vi "InitDir.vi"(8 "error in":errorcluster, 11 "MainFGV_data in":T1={"TestDir"=path "", "TestName"="", "task"="", "data_file"=refnum, "AcqQueue"=refnum, "StartTime"=timestamp(0 s since 1904-01-01), "config_channels"=[], "DAQmx Device"="", "Advanced"={"rate"=1652.0, "duration"=1.0, "thr"=100.0, "preTrigger"=100.0, "cutoff"=-3.0, "Filtro"=enum."Desativado", "highPass"=1000.0, "lowPass"=1000.0, "updateTime"=50.0}, "running"=FALSE, "hammerIndex"=0, "session"="localhost"} {"Advanced"."updateTime" format="%#_g ms"; "Advanced"."lowPass" format="%#_g Hz"; "Advanced"."highPass" format="%#_g Hz"; "Advanced"."cutoff" format="%#_g dB"; "Advanced"."preTrigger" format="%#_g ms"; "Advanced"."thr" format="%#_g N"; "Advanced"."duration" format="%#_g s"; "Advanced"."rate" min=1652.0 max=51200.0 format="%#_g Hz"}) -> (0 "error out":errorcluster, 3 "MainFGV_data":T1={"TestDir"=path "", "TestName"="", "task"="", "data_file"=refnum, "AcqQueue"=refnum, "StartTime"=timestamp(0 s since 1904-01-01), "config_channels"=[], "DAQmx Device"="", "Advanced"={"rate"=1652.0, "duration"=1.0, "thr"=100.0, "preTrigger"=100.0, "cutoff"=-3.0, "Filtro"=enum."Desativado", "highPass"=1000.0, "lowPass"=1000.0, "updateTime"=50.0}, "running"=FALSE, "hammerIndex"=0, "session"="localhost"} {"Advanced"."updateTime" format="%#_g ms"; "Advanced"."lowPass" format="%#_g Hz"; "Advanced"."highPass" format="%#_g Hz"; "Advanced"."cutoff" format="%#_g dB"; "Advanced"."preTrigger" format="%#_g ms"; "Advanced"."thr" format="%#_g N"; "Advanced"."duration" format="%#_g s"; "Advanced"."rate" min=1652.0 max=51200.0 format="%#_g Hz"})   [LabVIEW 2016]
uses:
  MainFGV_data.ctl
  Settings/config_board.ctl
  Settings/Advanced/AdvancedConfig.ctl
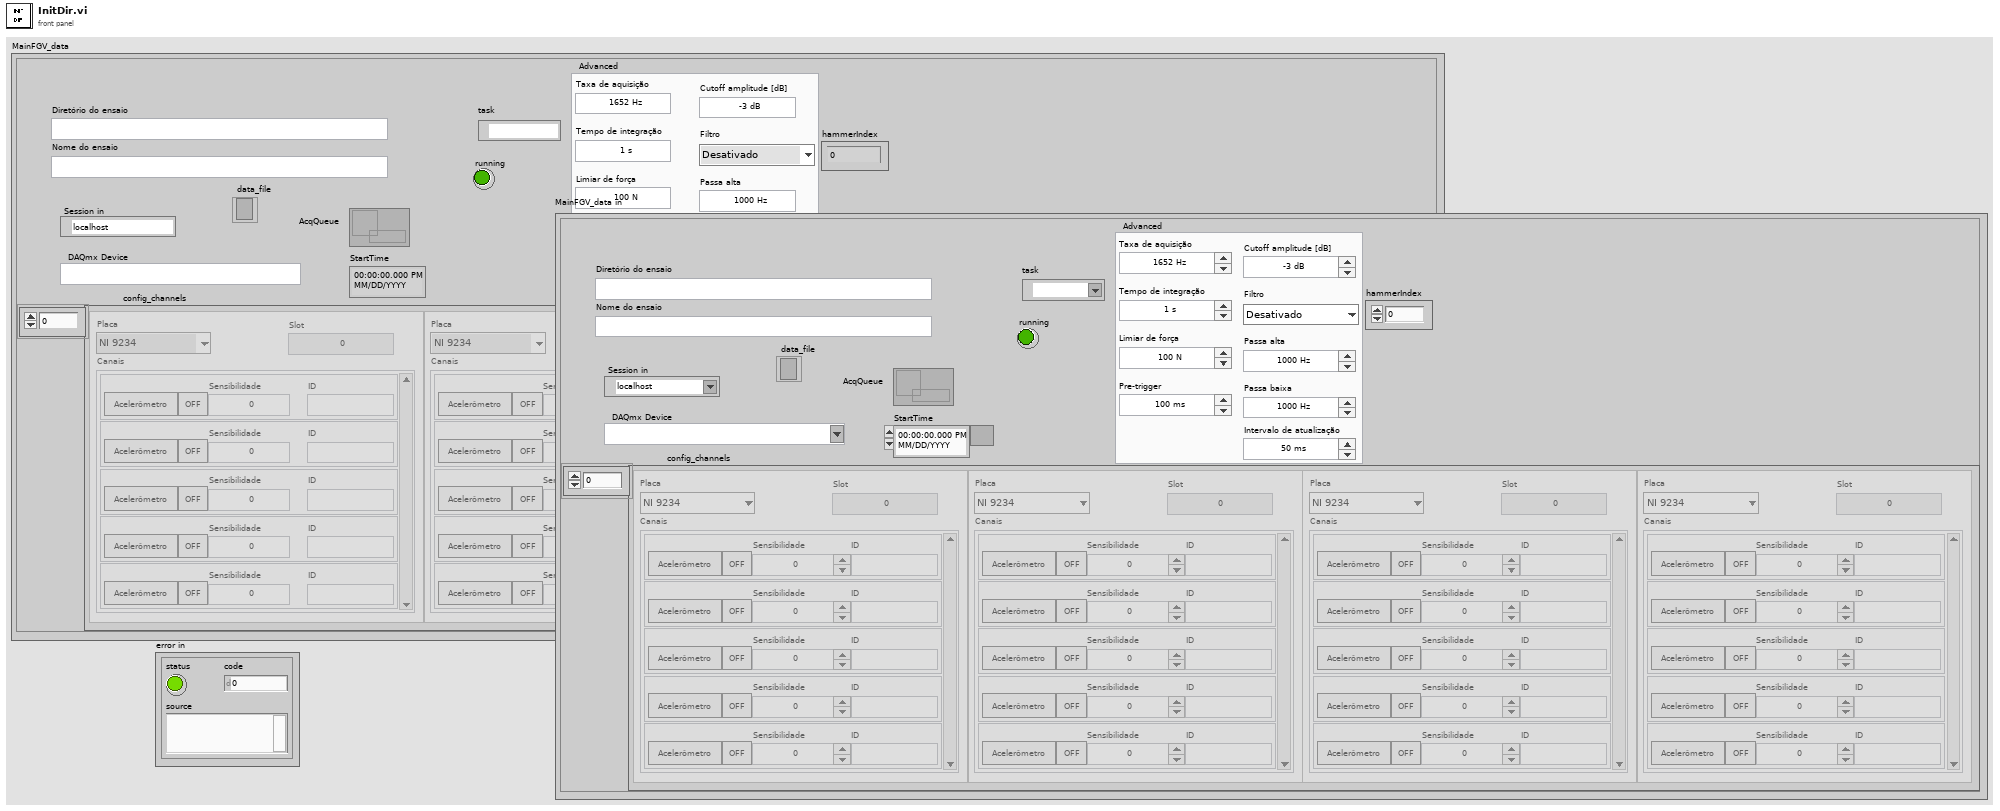
[diagram p1: front panel]
types:
  T1 = typedef "MainFGV_data.ctl" = cluster{"TestDir":path, "TestName":string, "task":refnum<k21>, "data_file":refnum<file>, "AcqQueue":refnum<queue>, "StartTime":timestamp, "config_channels":T2[], "DAQmx Device":tag, "Advanced":T3, "running":bool, "hammerIndex":i32, "session":refnum<k21>}
  T2 = typedef "config_board.ctl" = cluster{"board":enum16{"NI 9234", "NI 9205", "Não aplicável"}, "channels":cluster{"type":bool, "active":bool, "sens":dbl, "ID":string}[], "Slot":i32}
  T3 = typedef "AdvancedConfig.ctl" = cluster{"rate":dbl, "duration":dbl, "thr":dbl, "preTrigger":dbl, "cutoff":dbl, "Filtro":enum16{"Desativado", "Passa banda", "Passa alta", "Passa baixa"}, "highPass":dbl, "lowPass":dbl, "updateTime":dbl}
  T4 = enum16{"open", "replace", "create", "open or create", "replace or create", "replace or create with confirmation"}
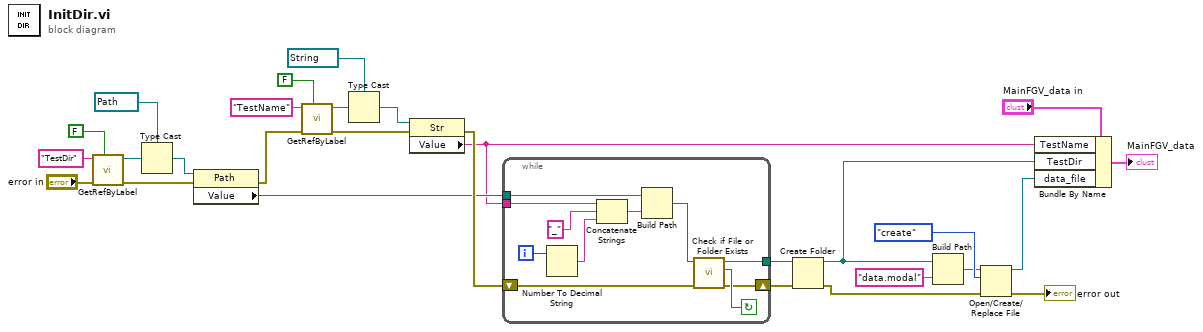
[diagram p0: block diagram]
diagram:
  n1 = call "GetRefByLabel.vi"("InsideTab"=FALSE, "error in"="error in", "Label"="TestDir") -> ("error out"=w8:errorcluster, "Ctl Refnum"=w12:refnum<vi>)  [unwired: 6 in, 1 out]
  n2 = Type Cast(type=refnum<vi> refnum ("TesrtDir"), x=w12) -> (*(type *) &x=w10:refnum<vi>)
  n3 = property class="Path"(reference=w10, error in=w8) -> (error out=w2:errorcluster, "Value"=w9:path)  [unwired: 1 out]
  n4 = call "GetRefByLabel.vi"("InsideTab"=FALSE, "error in"=w2, "Label"="TestName") -> ("error out"=w4:errorcluster, "Ctl Refnum"=w7:refnum<vi>)  [unwired: 6 in, 1 out]
  n5 = Type Cast(type=refnum<vi> refnum ("TestName"), x=w7) -> (*(type *) &x=w5:refnum<vi>)
  n6 = property class="Str"(reference=w5, error in=w4) -> (error out=w28:errorcluster, "Value"=w3:string)  [unwired: 1 out]
  n7 = while {
    tunnel: w3 -> [w38]
    tunnel: w9 -> [w36]
    shift-right: [w32] -> w27
    shift-left: w28 -> [w34]
    tunnel: [w31] -> w26
    i -> [w39]
    stop <- w33 continue-if-true
    n8 = Number To Decimal String(number=w39) -> (decimal integer string=w30:string)  [unwired: 1 in]
    n9 = Concatenate Strings(w38, "_" ("string"), w30) -> (w37:string)
    n10 = Build Path(base path=w36, name or relative path=w37) -> (appended path=w35:path)
    n11 = call <vilib>:"Check if File or Folder Exists.vi"("error in (no error)"=w34, "path"=w35) -> ("error out"=w32:errorcluster, "file or folder exists?"=w33:bool, "dup path"=w31:path)  [unwired: 7 in]
  }
  n12 = Create Folder(path (use dialog)=w26, error in=w27) -> (created path=w24:path, error out=w23:errorcluster)  [unwired: 1 in, 1 out]
  n13 = Build Path(base path=w24, name or relative path="data.modal") -> (appended path=w20:path)
  n14 = Open/Create/Replace File(file path (use dialog)=w20, error in=w23, operation (0:open)=T4."create") -> (refnum out=w19:refnum<file>, error out=→"error out":errorcluster)  [unwired: 3 in, 1 out]
  n15 = Bundle By Name(cluster="MainFGV_data in", "TestName"=w3, "TestDir"=w24, "data_file"=w19) -> (→"MainFGV_data":T1)
